vi "Write Messages.vi"(8 "error in (no error)":errorcluster, 10 "Messages":refnum<class "Registry.lvclass">, 11 "Minor Frame in":refnum<class "Minor Frame.lvclass">) -> (0 "error out":errorcluster, 3 "Minor Frame out":refnum<class "Minor Frame.lvclass">)   [LabVIEW 2020, in "BCI-1553 API.lvlib" / "Minor Frame.lvclass"]
uses:
  Minor Frame.lvclass
  Dependencies/Registry/Registry.lvclass
  Minor Frame.lvclass/Minor Frame.ctl
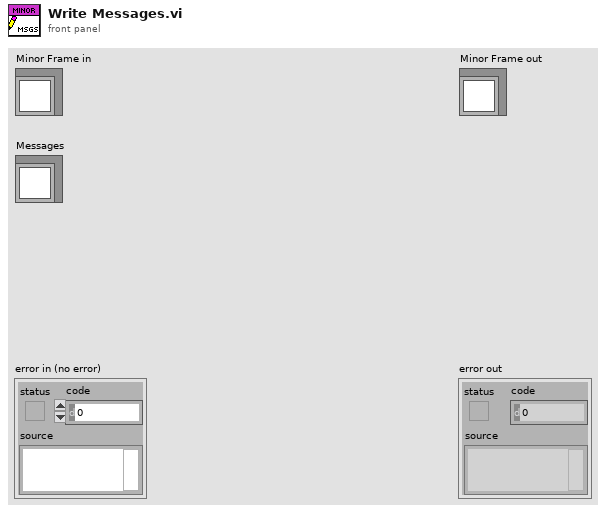
[diagram p1: front panel]
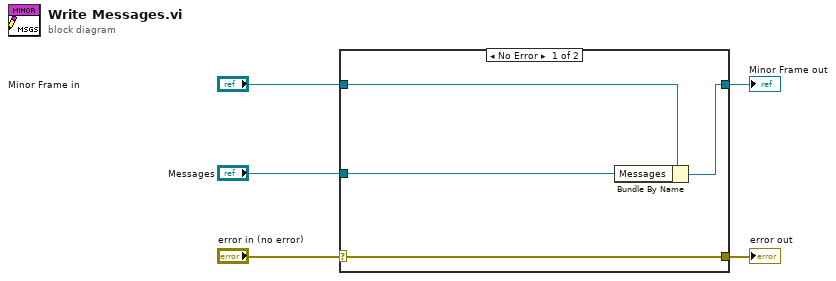
[diagram p0: block diagram]
diagram:
  n1 = case shown="No Error" "error in (no error)" {
    selector: "error in (no error)" -> [w9 w10]
    tunnel: [w9 w10] -> w4
    tunnel: [w7 w11] -> w2
    tunnel: "Minor Frame in" -> [w8 w11]
    tunnel: "Messages" -> [w6 _]
    frame No Error {
      n2 = Bundle By Name(cluster=w8, "Messages"=w6) -> (w7:refnum<class "Minor Frame.lvclass">)
    }
    frame Error {
    }
  }
  "error out" <- w4
  "Minor Frame out" <- w2
